vi "LoadUserInterface.vi"(8 "error in (no error)":errorcluster, 10 "Actor In":refnum<class "Actor.lvclass">, 11 "DataLogger in":refnum<class "DataLogger.lvclass">) -> (0 "error out":errorcluster, 3 "DataLogger out":refnum<class "DataLogger.lvclass">)   [LabVIEW 2020, in "DataLogger.lvlib" / "DataLogger.lvclass"]
uses:
  DataLogger.lvclass
  <vilib>/ActorFramework/Actor/Actor.lvclass
  DataLoggerUI/DataLoggerUI.lvclass
  C:/Program Files/National Instruments/LabVIEW 2020/vi.lib/ActorFramework/Actor/Actor.lvclass
  DataProcessor/DataProcessor/DataProcessor.lvclass
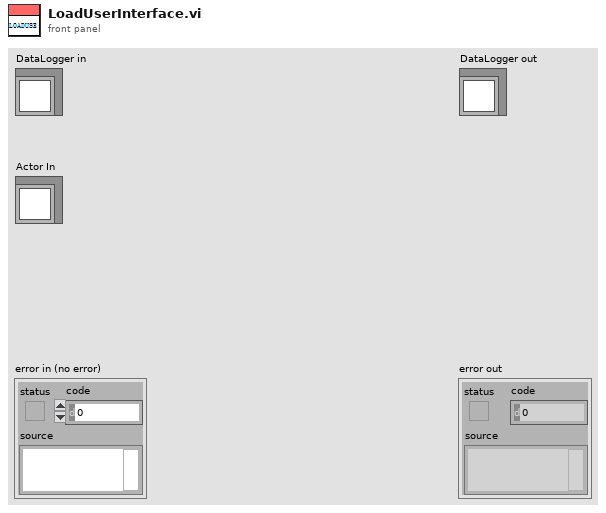
[diagram p1: front panel]
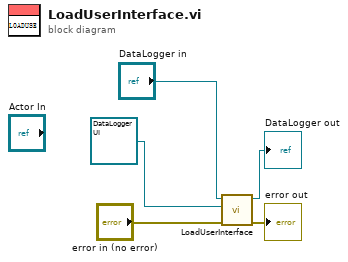
[diagram p0: block diagram]
diagram:
  n1 = call-parent "LoadUserInterface.vi"("error in (no error)"="error in (no error)", "Actor In"=refnum<class "DataLoggerUI.lvclass"> refnum ("DataLogger.lvlib:DataLoggerUI.lvclass"), "DataProcessor in"="DataLogger in") -> ("error out"=→"error out":errorcluster, "DataProcessor out"=→"DataLogger out":refnum<class "DataLogger.lvclass">)  [unwired: 7 in]
